vi "c Spark Destroy.vi"(8 "error in (no error)":errorcluster, 11 "handle":T1) -> (0 "error out":errorcluster, 3 "handle":T1)   [LabVIEW 2023, in "REVLibDriver.lvlib"]
doc: "void c_Spark_Destroy(c_Spark_handle handle);"
uses:
  REVLibDriver.lvlib
  REVLibDriver.dll
  Custom Controls/c_Spark_handle.ctl
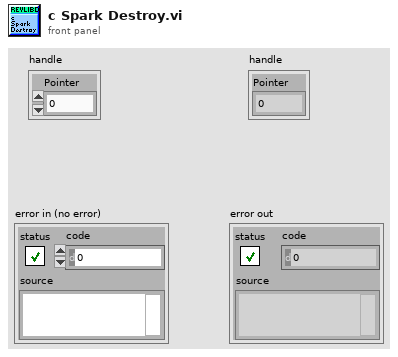
[diagram p1: front panel]
types:
  T1 = typedef "REVLibDriver.lvlib/c_Spark_handle.ctl" = cluster{"Pointer":u64}
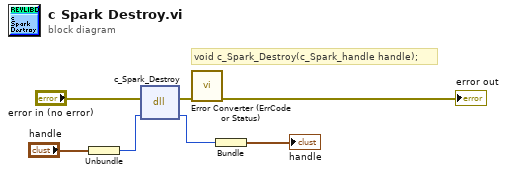
[diagram p0: block diagram]
diagram:
  # "void c_Spark_Destroy(c_Spark_handle handle);"
  n1 = Unbundle("handle") -> ("Pointer"=w2:u64)
  n2 = dll-call lib="REVLibDriver.*" fn="c_Spark_Destroy"(error in="error in (no error)", "handle"=w2) -> (error out=w4:errorcluster, "handle"=w6:u64)  [unwired: 3 in, 1 out]
  n3 = call "Error Converter (ErrCode or Status).vi"("error in (no error)"=w4) -> ("error out"=→"error out":errorcluster)  [unwired: 10 in]
  n4 = Bundle("handle"=w6) -> (→"handle":cluster{"handle":u64})  [unwired: 1 in]
